vi "Read Last contact.vi"(8 "error in (no error)":errorcluster, 11 "Server in":refnum<class "SLMServer.lvclass">) -> (0 "error out":errorcluster, 2 "Last contact":dbl[](array[numeric]), 3 "Server out":refnum<class "SLMServer.lvclass">)   [LabVIEW 2013, in "SLMServer.lvlib" / "SLMServer.lvclass"]
uses:
  SLMServer.lvclass
  SLMServer.lvclass/SLMServer.ctl
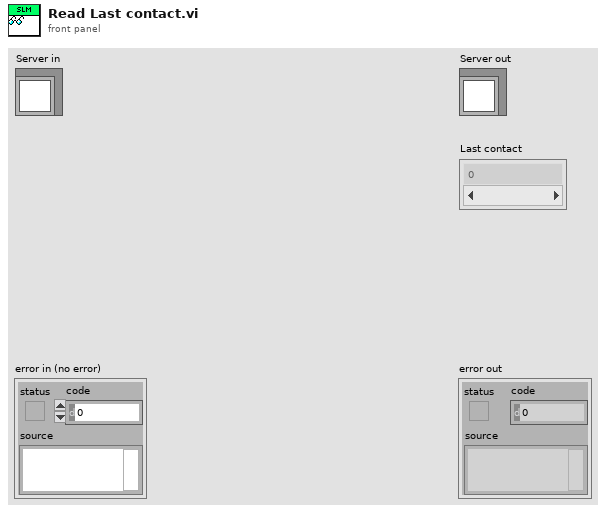
[diagram p1: front panel]
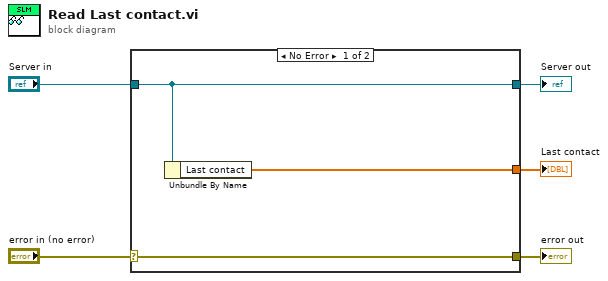
[diagram p0: block diagram]
diagram:
  n1 = case shown="No Error" "error in (no error)" {
    selector: "error in (no error)" -> [w8 w9]
    tunnel: [w8 w9] -> w4
    tunnel: [w7 w10] -> w2
    tunnel: "Server in" -> [w7 w10]
    tunnel: [w6 _] -> w1
    frame No Error {
      n2 = Unbundle By Name(w7) -> ("Last contact"=w6:dbl[])
    }
    frame Error {
    }
  }
  "error out" <- w4
  "Server out" <- w2
  "Last contact" <- w1
